vi "Begin.vi"(8 "error in":errorcluster) -> (0 "error out":errorcluster)   [LabVIEW 2017]
doc: "Called before other user functions, this VI is expected to open initial I/O refnums, load in file data, and do all program initialization. Notice that the <B>error out</B> terminal is simply used for data flow. Wiring it to other structures or subVIs ensures that this VI runs first."
uses:
  <vilib>/Rock Robotics/WPI/DriverStation/WPI_DriverStationRobotMode2.ctl
  <vilib>/Rock Robotics/WPI/Joystick/WPI_JoystickDeviceEnum.ctl
  <vilib>/Rock Robotics/WPI/Solenoid/WPI_SolenoidChannel.ctl
  <vilib>/Rock Robotics/WPI/ThirdParty/Sensors/navX/_TypeDefs/FRIC_navX_DeviceNumbersTypeDef.ctl
  <vilib>/Rock Robotics/SystemInterfaces/i2clib/i2c_bus.ctl
  Robot Global Data.vi
  <vilib>/Rock Robotics/Network Tables/NT Write String Array.vi
  <vilib>/Rock Robotics/WPI/Utilities/WPI_GetSetVariantRefNum.vi
  <vilib>/Rock Robotics/WPI/Solenoid/WPI_SolenoidOpenDouble.vi
  <vilib>/Rock Robotics/WPI/RobotDrive/WPI_RobotDriveOpen4MotorWithExistingMotors.vi
  <vilib>/Rock Robotics/WPI/RobotDrive/WPI_RobotDriveOpen2MotorWithExistingMotors.vi
  <vilib>/Rock Robotics/WPI/ThirdParty/Sensors/navX/_Processing Loop/FRIC_navX_Internal_I2C_ProcessingLoop.vi
  <vilib>/Rock Robotics/SystemInterfaces/AI/FPGA_AIChannel.ctl
  <vilib>/Rock Robotics/WPI/Ultrasonic/WPI_SonarMB1010AnalogRefNum Registry Set.vi
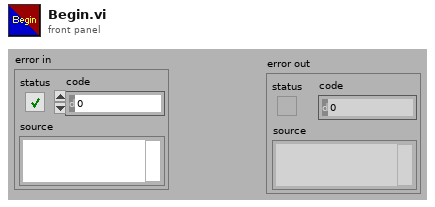
[diagram p1: front panel]
types:
  T1 = typedef "i2c_bus.ctl" = enum16{"I2C On-Board", "I2C MXP", "Invalid"}
  T2 = typedef "FRIC_navX_DeviceNumbersTypeDef.ctl" = enum16{"Dev0", "Dev1", "Dev2", "Dev3"}
  T3 = typedef "WPI_SolenoidChannel.ctl" = enum8{"Solenoid 0", "Solenoid 1", "Solenoid 2", "Solenoid 3", "Solenoid 4", "Solenoid 5", "Solenoid 6", "Solenoid 7", "Invalid"}
  T4 = typedef "WPI_JoystickDeviceEnum.ctl" = enum16{"USB 0", "USB 1", "USB 2", "USB 3", "USB 4", "USB 5"}
  T5 = typedef "WPI_DriverStationRobotMode2.ctl" = enum16{"Autonomous Disabled", "Autonomous Enabled", "Teleop Disabled", "Teleop Enabled", "Disconnected", "Finish", "Test Disabled", "Test Enabled", "Emergency Stopped"}
  T6 = typedef "WPI_MotorControlDeviceRef.ctl" = cluster{"DeviceStatus":errorcluster, "Type":T7, "PWM":cluster{"PWM Channel":T8, "DeadBand":T9}, "CAN":cluster{"Device Number":u8, "SetOutput VI Ref":variant, "GetOutput VI Ref":variant, "Enable VI Ref":variant, "Disable VI Ref":variant, "Data":variant}, "Invert":bool, "DIO PWM":cluster{"PWM \"Enable\" Channel":T8, "DIOChannel":T10, "PWM Rate":dbl}}
  T7 = typedef "WPI_MotorControlType.ctl" = enum16{"PWM", "CAN", "DIO PWM"}
  T8 = typedef "FPGA_DIOPWMChannel.ctl" = enum8{"PWM 0", "PWM 1", "PWM 2", "PWM 3", "PWM 4", "PWM 5", "PWM 6", "PWM 7", "PWM 8", "PWM 9", "PWM MXP 0", "PWM MXP 1", "PWM MXP 2", "PWM MXP 3", "PWM MXP 4", "PWM MXP 5", "PWM MXP 6", "PWM MXP 7", "PWM MXP 8", "PWM MXP 9", "Invalid"}
  T9 = typedef "WPI_PWMDeadband.ctl" = cluster{"Name":string, "maxPositivePwm":i32, "minPositivePwm":i32, "centerPwm":i32, "maxNegativePwm":i32, "minNegativePwm":i32, "angularRange":u16}
  T10 = typedef "FPGA_DIOChannel.ctl" = enum8{"DIO 0", "DIO 1", "DIO 2", "DIO 3", "DIO 4", "DIO 5", "DIO 6", "DIO 7", "DIO 8", "DIO 9", "DIO MXP 0", "DIO MXP 1", "DIO MXP 2", "DIO MXP 3", "DIO MXP 4", "DIO MXP 5", "DIO MXP 6", "DIO MXP 7", "DIO MXP 8", "DIO MXP 9", "DIO MXP 10", "DIO MXP 11", "DIO MXP 12", "DIO MXP 13", "DIO MXP 14", "DIO MXP 15", "SPI Port CS1", "SPI Port CS2", "SPI Port CS3", "SPI Port MISO", "SPI Port MOSI", "Invalid"}
  T11 = typedef "FPGA_AIChannel.ctl" = enum8{"AI 0", "AI 1", "AI 2", "AI 3", "AI MXP 0", "AI MXP 1", "AI MXP 2", "AI MXP 3", "Invalid"}
  T12 = typedef "WPI_SonarMB1010AnalogDeviceRef.ctl" = cluster{"AIDeviceRef":T13, "Scaling factor (V/in)":dbl, "Average Bits":u8}
  T13 = typedef "WPI_AnalogChannelDevRef.ctl" = cluster{"DevStatus":errorcluster, "Analog Channel":T11}
  T14 = typedef "WPI_CompressorDevRef.ctl" = cluster{"DevStatus":errorcluster, "Pneumatics Control Module":u8}
  T15 = typedef "WPI_JoystickDevRef.ctl" = cluster{"Device":T4}
  T16 = typedef "WPI_RobotDriveDevRef.ctl" = cluster{"DevStatus":errorcluster, "Motors[]":T6[], "Square Inputs":bool, "Max Output":dbl}
  T17 = typedef "WPI_SolenoidDevRef.ctl" = cluster{"DevStatus":errorcluster, "Pneumatics Control Module":u8, "Forward Solenoid Channel":T3, "Reverse Solenoid Channel":T3}
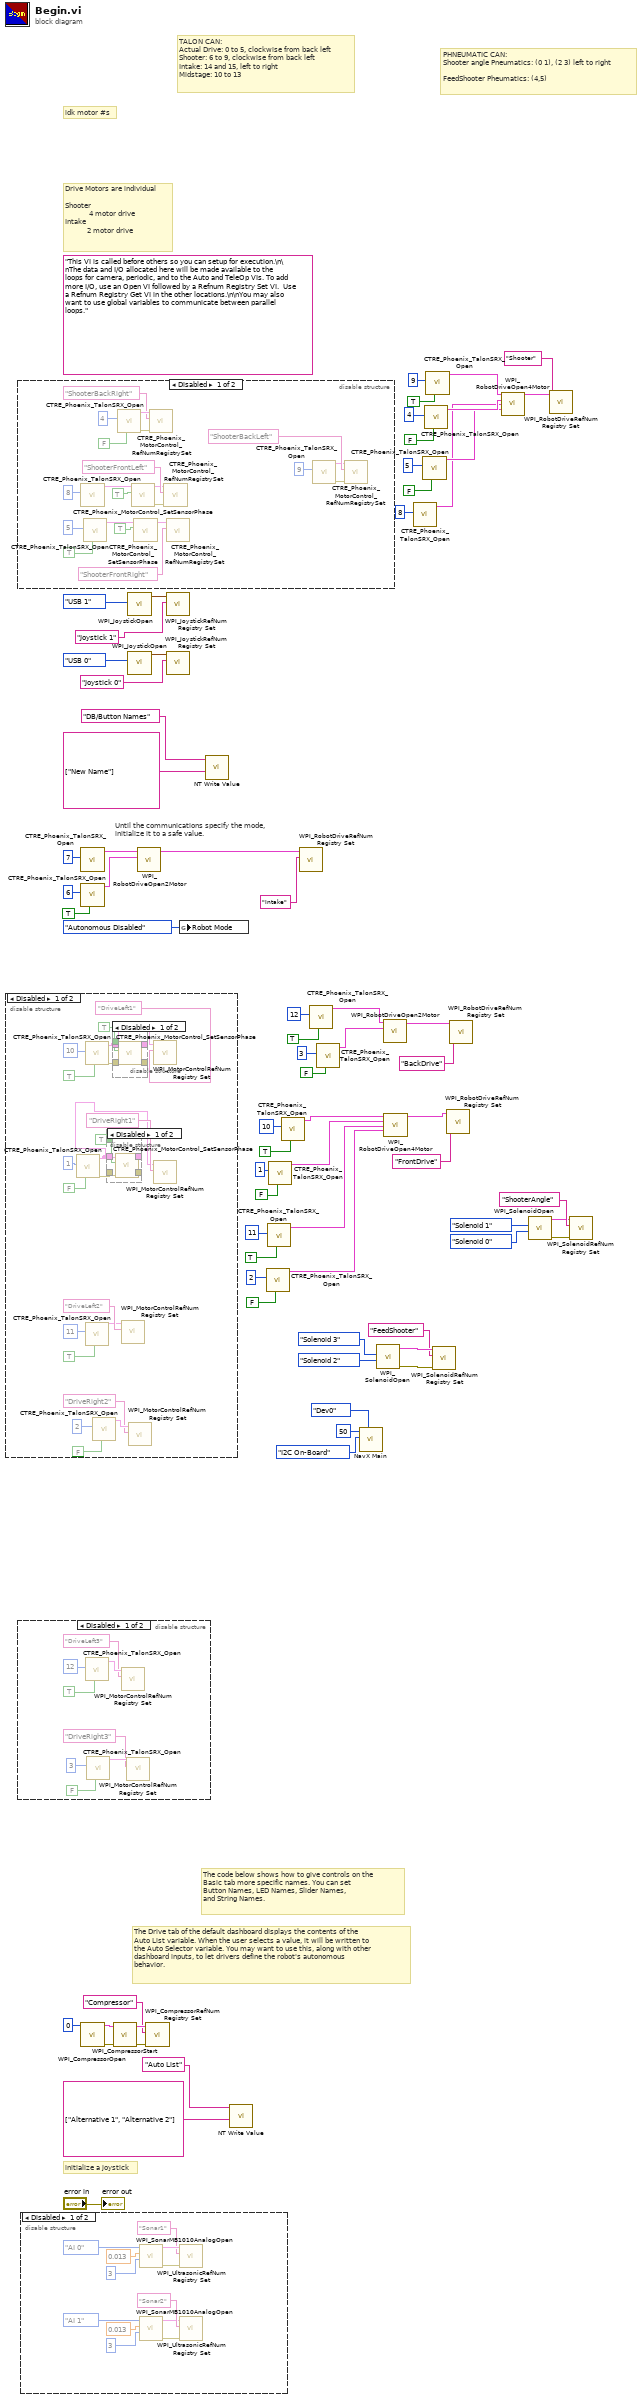
[diagram p0: block diagram]
diagram:
  (unwired) "This VI is called before others so you can setup for execution.\n\nThe data and I/O allocated here will be made available to the loops for camera, periodic, and to the Auto and TeleOp VIs. To add more I/O, use an Open VI followed by a Refnum Registry Set VI.  Use a Refnum Registry Get VI in the other locations.\n\nYou may also want to use global variables to communicate between parallel loops."
  # "Until the communications specify the mode,\ninitialize it to a safe value."
  # "idk motor #s"
  # "Drive Motors are individual\n\nShooter \n            4 motor drive\nIntake\n           2 motor drive"
  # "PHNEUMATIC CAN:\nShooter angle Pneumatics: (0 1), (2 3) left to right\n\nFeedShooter Pheumatics: (4,5)"
  # "TALON CAN: \nActual Drive: 0 to 5, clockwise from back left\nShooter: 6 to 9, clockwise from back left\nIntake: 14 and 15, left to right\nMidstage: 10 to 13"
  # "The Drive tab of the default dashboard displays the contents of the\nAuto List variable. When the user selects a value, it will be written to\nthe Auto Selector variable. You may want to use this, along with other\ndashboard inputs, to let drivers define the robot's autonomous\nbehavior."
  # "The code below shows how to give controls on the\nBasic tab more specific names. You can set\nButton Names, LED Names, Slider Names,\nand String Names."
  # "initialize a joystick"
  n1 = disable-structure shown="Disabled" {
    frame Disabled {
      n2 = call <vilib>:"CTRE_Phoenix_TalonSRX_Open.vi"("Invert"=FALSE, "Device Number"=u8 1) -> ("error out"=w84:errorcluster, "CAN Talon SRX Ref"=w74:T6)  [unwired: 8 in]
      n3 = call <vilib>:"CTRE_Phoenix_TalonSRX_Open.vi"("Invert"=TRUE, "Device Number"=u8 10) -> ("error out"=w83:errorcluster, "CAN Talon SRX Ref"=w75:T6)  [unwired: 8 in]
      n4 = call <vilib>:"CTRE_Phoenix_TalonSRX_Open.vi"("Invert"=TRUE, "Device Number"=u8 11) -> ("CAN Talon SRX Ref"=w78:T6)  [unwired: 8 in, 1 out]
      n5 = call <vilib>:"CTRE_Phoenix_TalonSRX_Open.vi"("Invert"=FALSE, "Device Number"=u8 2) -> ("CAN Talon SRX Ref"=w81:T6)  [unwired: 8 in, 1 out]
      n6 = disable-structure shown="Disabled" {
        disable-tunnel: w74 -> [w103 _]
        disable-tunnel: TRUE ("PhaseSensor") -> [w102 _]
        disable-tunnel: w84 -> [w101 _]
        disable-tunnel: [w100 _] -> _
        disable-tunnel: [w99 _] -> _
        frame Disabled {
          n7 = call <vilib>:"CTRE_Phoenix_MotorControl_SetSensorPhase.vi"("error in (no error)"=w101, "PhaseSensor"=w102, "PhoenixMotorControlDevRef"=w103) -> ("error out"=w99:errorcluster, "PhoenixMotorControlDevRef"=w100:T6)  [unwired: 7 in]
        }
        frame Enabled {
        }
      }
      n8 = disable-structure shown="Disabled" {
        disable-tunnel: w75 -> [w98 _]
        disable-tunnel: [w97 _] -> _
        disable-tunnel: w83 -> [w96 _]
        disable-tunnel: [w95 _] -> _
        disable-tunnel: TRUE ("PhaseSensor") -> [w94 _]
        frame Disabled {
          n9 = call <vilib>:"CTRE_Phoenix_MotorControl_SetSensorPhase.vi"("error in (no error)"=w96, "PhaseSensor"=w94, "PhoenixMotorControlDevRef"=w98) -> ("error out"=w95:errorcluster, "PhoenixMotorControlDevRef"=w97:T6)  [unwired: 7 in]
        }
        frame Enabled {
        }
      }
      n10 = call <vilib>:"WPI_MotorControlRefNum Registry Set.vi"("refnum name"="DriveLeft2", "MotorControlDevRef"=w78) -> ()  [unwired: 8 in, 2 out]
      n11 = call <vilib>:"WPI_MotorControlRefNum Registry Set.vi"("refnum name"="DriveRight2", "MotorControlDevRef"=w81) -> ()  [unwired: 8 in, 2 out]
      n12 = call <vilib>:"WPI_MotorControlRefNum Registry Set.vi"("refnum name"="DriveLeft1", "MotorControlDevRef"=w75) -> ()  [unwired: 8 in, 2 out]
      n13 = call <vilib>:"WPI_MotorControlRefNum Registry Set.vi"("refnum name"="DriveRight1", "MotorControlDevRef"=w74) -> ()  [unwired: 8 in, 2 out]
    }
    frame Enabled {
    }
  }
  n14 = disable-structure shown="Disabled" {
    frame Disabled {
      n15 = call <vilib>:"CTRE_Phoenix_TalonSRX_Open.vi"("Device Number"=u8 8) -> ("CAN Talon SRX Ref"=w109:T6)  [unwired: 9 in, 1 out]
      n16 = call <vilib>:"CTRE_Phoenix_TalonSRX_Open.vi"("Invert"=TRUE, "Device Number"=u8 5) -> ("CAN Talon SRX Ref"=w107:T6)  [unwired: 8 in, 1 out]
      n17 = call <vilib>:"CTRE_Phoenix_TalonSRX_Open.vi"("Invert"=FALSE, "Device Number"=u8 4) -> ("error out"=w114:errorcluster, "CAN Talon SRX Ref"=w118:T6)  [unwired: 8 in]
      n18 = call <vilib>:"CTRE_Phoenix_MotorControl_SetSensorPhase.vi"("PhaseSensor"=TRUE, "PhoenixMotorControlDevRef"=w109) -> ("error out"=w110:errorcluster, "PhoenixMotorControlDevRef"=w108:T6)  [unwired: 8 in]
      n19 = call <vilib>:"CTRE_Phoenix_MotorControl_SetSensorPhase.vi"("PhaseSensor"=TRUE, "PhoenixMotorControlDevRef"=w107) -> ("PhoenixMotorControlDevRef"=w106:T6)  [unwired: 8 in, 1 out]
      n20 = call <vilib>:"CTRE_Phoenix_MotorControl_RefNumRegistrySet.vi"("error in (no error)"=w114, "refnum name"="ShooterBackRight", "PhoenixMotorControlDevRef"=w118) -> ()  [unwired: 7 in, 2 out]
      n21 = call <vilib>:"CTRE_Phoenix_MotorControl_RefNumRegistrySet.vi"("error in (no error)"=w110, "refnum name"="ShooterFrontLeft", "PhoenixMotorControlDevRef"=w108) -> ()  [unwired: 7 in, 2 out]
      n22 = call <vilib>:"CTRE_Phoenix_MotorControl_RefNumRegistrySet.vi"("refnum name"="ShooterFrontRight", "PhoenixMotorControlDevRef"=w106) -> ()  [unwired: 8 in, 2 out]
      n23 = call <vilib>:"CTRE_Phoenix_TalonSRX_Open.vi"("Device Number"=u8 9) -> ("error out"=w113:errorcluster, "CAN Talon SRX Ref"=w121:T6)  [unwired: 9 in]
      n24 = call <vilib>:"CTRE_Phoenix_MotorControl_RefNumRegistrySet.vi"("error in (no error)"=w113, "refnum name"="ShooterBackLeft", "PhoenixMotorControlDevRef"=w121) -> ()  [unwired: 7 in, 2 out]
    }
    frame Enabled {
    }
  }
  n25 = disable-structure shown="Disabled" {
    frame Disabled {
      n26 = call <vilib>:"CTRE_Phoenix_TalonSRX_Open.vi"("Invert"=TRUE, "Device Number"=u8 12) -> ("CAN Talon SRX Ref"=w126:T6)  [unwired: 8 in, 1 out]
      n27 = call <vilib>:"CTRE_Phoenix_TalonSRX_Open.vi"("Invert"=FALSE, "Device Number"=u8 3) -> ("CAN Talon SRX Ref"=w128:T6)  [unwired: 8 in, 1 out]
      n28 = call <vilib>:"WPI_MotorControlRefNum Registry Set.vi"("refnum name"="DriveLeft3", "MotorControlDevRef"=w126) -> ()  [unwired: 8 in, 2 out]
      n29 = call <vilib>:"WPI_MotorControlRefNum Registry Set.vi"("refnum name"="DriveRight3", "MotorControlDevRef"=w128) -> ()  [unwired: 8 in, 2 out]
    }
    frame Enabled {
    }
  }
  n30 = disable-structure shown="Disabled" {
    frame Disabled {
      n31 = call <vilib>:"WPI_SonarMB1010AnalogOpen.vi"("Average Bits"=u8 3, "Scaling factor (V/in)"=0.013, "Analog Channel"=FPGA_AIChannel."AI 0") -> ("error out"=w143:errorcluster, "SonarMB1010AnalogDevRef"=w142:T12)  [unwired: 7 in]
      n32 = call <vilib>:"WPI_SonarMB1010AnalogOpen.vi"("Average Bits"=u8 3, "Scaling factor (V/in)"=0.013, "Analog Channel"=FPGA_AIChannel."AI 1") -> ("error out"=w138:errorcluster, "SonarMB1010AnalogDevRef"=w139:T12)  [unwired: 7 in]
      n33 = call-poly <vilib>:"WPI_UltrasonicRefNum Registry Set.vi"("error in (no error)"=w143, "refnum name"="Sonar1", "SonarMB1010AnalogDevRef"=w142) -> ()  [unwired: 7 in, 2 out]
      n34 = call-poly <vilib>:"WPI_UltrasonicRefNum Registry Set.vi"("error in (no error)"=w138, "refnum name"="Sonar2", "SonarMB1010AnalogDevRef"=w139) -> ()  [unwired: 7 in, 2 out]
    }
    frame Enabled {
    }
  }
  n35 = call <vilib>:"CTRE_Phoenix_TalonSRX_Open.vi"("Device Number"=u8 7) -> ("CAN Talon SRX Ref"=w23:T6)  [unwired: 9 in, 1 out]
  n36 = call <vilib>:"CTRE_Phoenix_TalonSRX_Open.vi"("Invert"=TRUE, "Device Number"=u8 6) -> ("CAN Talon SRX Ref"=w20:T6)  [unwired: 8 in, 1 out]
  n37 = call <vilib>:"WPI_CompressorOpen.vi"("Pneumatics Control Module (0)"=u8 0) -> ("CompressorDevRef"=w65:T14, "error out"=w63:errorcluster)  [unwired: 13 in]
  n38 = call <vilib>:"WPI_CompressorStart.vi"("error in (no error)"=w63, "CompressorDevRef"=w65) -> ("error out"=w62:errorcluster, "CompressorDevRef"=w64:T14)  [unwired: 8 in]
  n39 = call <vilib>:"WPI_JoystickOpen.vi"("JoystickDevice"=WPI_JoystickDeviceEnum."USB 1") -> ("JoystickDevRef"=w53:T15)  [unwired: 10 in]
  n40 = call <vilib>:"WPI_JoystickOpen.vi"("JoystickDevice"=WPI_JoystickDeviceEnum."USB 0") -> ("JoystickDevRef"=w73:T15)  [unwired: 10 in]
  n41 = call-poly <vilib>:"WPI_RobotDriveOpen2Motor.vi"("Right Motor Dev Ref"=w20, "Left Motor Dev Ref"=w23) -> ("RobotDriveDevRef"=w22:T16)  [unwired: 8 in, 1 out]
  n42 = call <vilib>:"WPI_CompressorRefNum Registry Set.vi"("error in (no error)"=w62, "refnum name"="Compressor", "CompressorDevRef"=w64) -> ()  [unwired: 7 in, 2 out]
  n43 = call <vilib>:"WPI_JoystickRefNum Registry Set.vi"("refnum name"="Joystick 1", "JoystickDevRef"=w53) -> ()  [unwired: 8 in, 2 out]
  n44 = call <vilib>:"WPI_JoystickRefNum Registry Set.vi"("refnum name"="Joystick 0", "JoystickDevRef"=w73) -> ()  [unwired: 8 in, 2 out]
  n45 = global write "Robot Global Data.vi" "Robot Mode"(WPI_DriverStationRobotMode2."Autonomous Disabled" ("Robot Mode")) -> ()
  n46 = call-poly <vilib>:"NT Write Value.vi"("String Array"=string[] ["New Name"], "Name"="DB/Button Names") -> ()  [unwired: 9 in, 1 out]
  n47 = call-poly <vilib>:"NT Write Value.vi"("String Array"=string[] ["Alternative 1", "Alternative 2"], "Name"="Auto List") -> ()  [unwired: 9 in, 1 out]
  n48 = call <vilib>:"CTRE_Phoenix_TalonSRX_Open.vi"("Invert"=FALSE, "Device Number"=u8 2) -> ("CAN Talon SRX Ref"=w36:T6)  [unwired: 8 in, 1 out]
  n49 = call <vilib>:"CTRE_Phoenix_TalonSRX_Open.vi"("Invert"=TRUE, "Device Number"=u8 11) -> ("CAN Talon SRX Ref"=w39:T6)  [unwired: 8 in, 1 out]
  n50 = call <vilib>:"CTRE_Phoenix_TalonSRX_Open.vi"("Invert"=FALSE, "Device Number"=u8 1) -> ("CAN Talon SRX Ref"=w42:T6)  [unwired: 8 in, 1 out]
  n51 = call <vilib>:"CTRE_Phoenix_TalonSRX_Open.vi"("Invert"=TRUE, "Device Number"=u8 10) -> ("CAN Talon SRX Ref"=w45:T6)  [unwired: 8 in, 1 out]
  n52 = call <vilib>:"WPI_RobotDriveRefNum Registry Set.vi"("refnum name"="Intake", "RobotDriveDevRef"=w22) -> ()  [unwired: 8 in, 2 out]
  n53 = call <vilib>:"CTRE_Phoenix_TalonSRX_Open.vi"("Invert"=TRUE, "Device Number"=u8 12) -> ("CAN Talon SRX Ref"=w33:T6)  [unwired: 8 in, 1 out]
  n54 = call <vilib>:"CTRE_Phoenix_TalonSRX_Open.vi"("Invert"=FALSE, "Device Number"=u8 3) -> ("CAN Talon SRX Ref"=w30:T6)  [unwired: 8 in, 1 out]
  n55 = call-poly <vilib>:"NavX Main.vi"("Device Number"=FRIC_navX_DeviceNumbersTypeDef."Dev0", "I2C Bus"=i2c_bus."I2C On-Board", "Rate (4Hz-200Hz)"=u8 50) -> ()  [unwired: 9 in]
  n56 = call-poly <vilib>:"WPI_SolenoidOpen.vi"("Reverse Solenoid Channel"=WPI_SolenoidChannel."Solenoid 2", "Forward Solenoid Channel"=WPI_SolenoidChannel."Solenoid 3") -> ("error out"=w51:errorcluster, "SolenoidDevRef"=w52:T17)  [unwired: 8 in]
  n57 = call-poly <vilib>:"WPI_RobotDriveOpen2Motor.vi"("Right Motor Dev Ref"=w30, "Left Motor Dev Ref"=w33) -> ("RobotDriveDevRef"=w29:T16)  [unwired: 8 in, 1 out]
  n58 = call-poly <vilib>:"WPI_RobotDriveOpen4Motor.vi"("Rear Left Motor Dev Ref"=w45, "Rear Right Motor Dev Ref"=w42, "Front Left Motor Dev Ref"=w39, "Front Right Motor Dev Ref"=w36) -> ("RobotDriveDevRef"=w27:T16)  [unwired: 10 in, 1 out]
  n59 = call <vilib>:"CTRE_Phoenix_TalonSRX_Open.vi"("Device Number"=u8 8) -> ("CAN Talon SRX Ref"=w7:T6)  [unwired: 9 in, 1 out]
  n60 = call <vilib>:"CTRE_Phoenix_TalonSRX_Open.vi"("Invert"=FALSE, "Device Number"=u8 5) -> ("CAN Talon SRX Ref"=w9:T6)  [unwired: 8 in, 1 out]
  n61 = call <vilib>:"CTRE_Phoenix_TalonSRX_Open.vi"("Invert"=FALSE, "Device Number"=u8 4) -> ("CAN Talon SRX Ref"=w16:T6)  [unwired: 8 in, 1 out]
  n62 = call <vilib>:"CTRE_Phoenix_TalonSRX_Open.vi"("Invert"=TRUE, "Device Number"=u8 9) -> ("CAN Talon SRX Ref"=w14:T6)  [unwired: 8 in, 1 out]
  n63 = call <vilib>:"WPI_SolenoidRefNum Registry Set.vi"("error in (no error)"=w51, "refnum name"="FeedShooter", "SolenoidDevRef"=w52) -> ()  [unwired: 7 in, 2 out]
  n64 = call <vilib>:"WPI_RobotDriveRefNum Registry Set.vi"("refnum name"="FrontDrive", "RobotDriveDevRef"=w27) -> ()  [unwired: 8 in, 2 out]
  n65 = call <vilib>:"WPI_RobotDriveRefNum Registry Set.vi"("refnum name"="BackDrive", "RobotDriveDevRef"=w29) -> ()  [unwired: 8 in, 2 out]
  n66 = call-poly <vilib>:"WPI_RobotDriveOpen4Motor.vi"("Rear Left Motor Dev Ref"=w14, "Rear Right Motor Dev Ref"=w16, "Front Left Motor Dev Ref"=w7, "Front Right Motor Dev Ref"=w9) -> ("RobotDriveDevRef"=w19:T16)  [unwired: 10 in, 1 out]
  n67 = call-poly <vilib>:"WPI_SolenoidOpen.vi"("Reverse Solenoid Channel"=WPI_SolenoidChannel."Solenoid 0", "Forward Solenoid Channel"=WPI_SolenoidChannel."Solenoid 1") -> ("error out"=w58:errorcluster, "SolenoidDevRef"=w57:T17)  [unwired: 8 in]
  n68 = call <vilib>:"WPI_RobotDriveRefNum Registry Set.vi"("refnum name"="Shooter", "RobotDriveDevRef"=w19) -> ()  [unwired: 8 in, 2 out]
  n69 = call <vilib>:"WPI_SolenoidRefNum Registry Set.vi"("error in (no error)"=w58, "refnum name"="ShooterAngle", "SolenoidDevRef"=w57) -> ()  [unwired: 7 in, 2 out]
  "error out" <- "error in"
